vi "write_ss_with_header.vi"(0 "Header String":string, 7 "Data to Write":dbl[][](array[numeric]) format="%.2f", 11 "Transpose Data?":bool, 13 "file (use dialog)":path, 14 "Error in":errorcluster) -> ()   [LabVIEW 2016]
doc: "Writes a text header and a 2D array to a file from the path output.\n\nThe parser string is [CR, CR, DDD, CR, CR].\n\nMuhannad Alghamdi\nPhysics 350"
uses:
  <vilib>/Utility/file.llb/Write Delimited Spreadsheet (DBL).vi
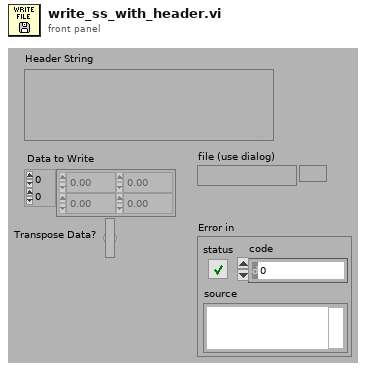
[diagram p1: front panel]
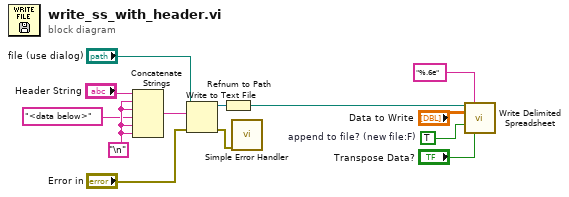
[diagram p0: block diagram]
diagram:
  w7 = TRUE  # append to file? (new file:F)
  w9 = "\n"
  n1 = Concatenate Strings("Header String", w9, w9, "<data below>", w9, w9) -> (w6:string)
  n2 = Write to Text File(file (use dialog)="file (use dialog)", text=w6, error in="Error in") -> (refnum out=w5:refnum<file>, error out=w3:errorcluster)  [unwired: 1 in, 1 out]
  n3 = Refnum to Path(1:w5) -> (0:w4:path)
  n4 = call <vilib>:"Simple Error Handler.vi"("error in (no error)"=w3) -> ()  [unwired: 4 in, 5 out]
  n5 = call-poly <vilib>:"Write Delimited Spreadsheet.vi"("file path (dialog if empty)"=w4, "format (%.3f)"="%.6e", "2D data"="Data to Write", "append to file? (new file:F)"=w7, "transpose? (no:F)"="Transpose Data?") -> ()  [unwired: 9 in, 2 out]
